vi "19052 Get_test_TIME.vi"(7 "Mode":T1, 8 "error in (no error)":errorcluster, 9 "Step":u16=1 min=1 max=99 step=1, 11 "VISA resource in":refnum<visa-resource-name>) -> (0 "error out":errorcluster, 1 "Test TIME":dbl format="%.1p", 3 "VISA resource out":refnum<visa-resource-name>)   [LabVIEW 2015]
uses:
  Type Definitions/ac_dc_ir_control.ctl
panel:
  out "output command":string
  # "Get test TIME"
  # "[s]"
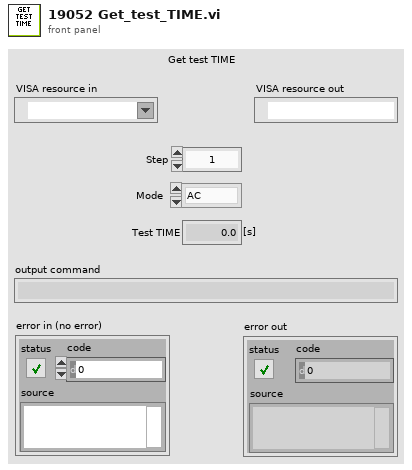
[diagram p1: front panel]
types:
  T1 = typedef "ac_dc_ir_control.ctl" = enum16{"AC", "DC", "IR"}
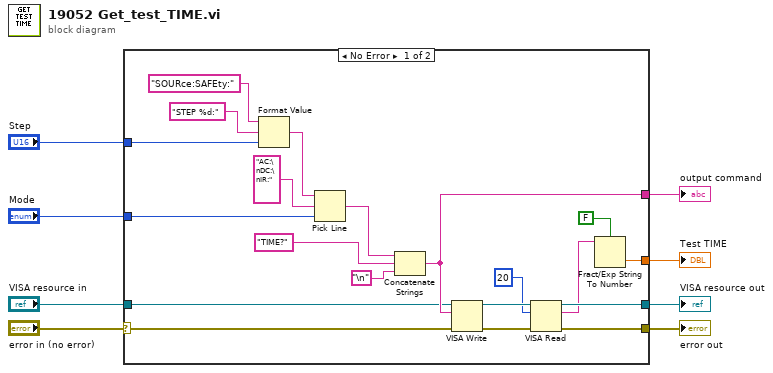
[diagram p0: block diagram]
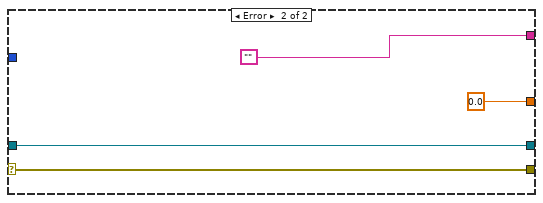
[diagram p2: hidden frame]
diagram:
  n1 = case shown="No Error" "error in (no error)" {
    selector: "error in (no error)" -> [w28 w32]
    tunnel: [w19 w32] -> w8
    tunnel: [w16 ""] -> w6
    tunnel: [w15 w30] -> w5
    tunnel: "Step" -> [w14 _]
    tunnel: "Mode" -> [w13 _]
    tunnel: "VISA resource in" -> [w12 w30]
    tunnel: [w10 0.0] -> w1
    frame No Error {
      n2 = Format Value(string ("")="SOURce:SAFEty:", format string="STEP %d:", value (0)=w14) -> (output string=w25:string)
      n3 = Pick Line(string ("")=w25, multi-line string="AC:\nDC:\nIR:", line index=w13) -> (output string=w21:string)
      n4 = Concatenate Strings(w21, "TIME?", "\n") -> (w16:string)
      n5 = VISA Write(VISA resource name=w12, write buffer=w16, error in (no error)=w28) -> (VISA resource name out=w18:refnum<visa-resource-name>, error out=w20:errorcluster)  [unwired: 1 out]
      n6 = VISA Read(VISA resource name=w18, byte count=u32 20, error in (no error)=w20) -> (VISA resource name out=w15:refnum<visa-resource-name>, read buffer=w11:string, error out=w19:errorcluster)  [unwired: 1 out]
      n7 = Fract/Exp String To Number(use system decimal point (T)=FALSE, string=w11) -> (number=w10:dbl)  [unwired: 2 in, 1 out]
    }
    frame Error {
    }
  }
  "error out" <- w8
  "VISA resource out" <- w5
  "output command" <- w6
  "Test TIME" <- w1
